vi "LinearSystemLoop_DiffDrv_Pack_Ctrl.vi"(4 "Max Control Effort":dbl=12.0, 6 "Right Vel Ctrl Tol m/s":dbl=0.04, 7 "Left Vel Model Std Dev m/s":dbl=0.1, 8 "Left Vel Ctrl Tol m/s":dbl=0.04, 9 "Right Vel Meas Std Dev m/s":dbl=0.03, 10 "Left Vel Meas Std Dev m/s":dbl=0.03, 11 "Right Vel Model Std Dev m/s":dbl=0.1) -> (3 "LinearSystemLoop_DiffDrv_Ctrl_Params":T1={"Left Vel Model Std Dev m/s"=0.0, "Left Vel Meas Std Dev m/s"=0.0, "Left Vel Ctrl Tol m/s"=0.0, "Max Control Effort"=0.0, "Right Vel Ctrl Tol m/s"=0.8, "Right Vel Meas Std Dev m/s"=0.02, "Right Vel Model Std Dev m/s"=0.0})   [LabVIEW 2019, in "Trajectory_Library.lvlib"]
uses:
  Trajectory_Library.lvlib
  TypeDef/LINEAR_SYSTEM_LOOP_DIFF_DRV_CTRL_PARAMS.CTL
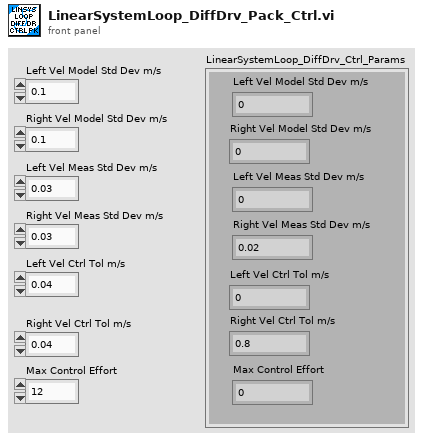
[diagram p1: front panel]
types:
  T1 = typedef "Trajectory_Library.lvlib/LINEAR_SYSTEM_LOOP_DIFF_DRV_CTRL_PARAMS.CTL" = cluster{"Left Vel Model Std Dev m/s":dbl, "Left Vel Meas Std Dev m/s":dbl, "Left Vel Ctrl Tol m/s":dbl, "Max Control Effort":dbl, "Right Vel Ctrl Tol m/s":dbl, "Right Vel Meas Std Dev m/s":dbl, "Right Vel Model Std Dev m/s":dbl}
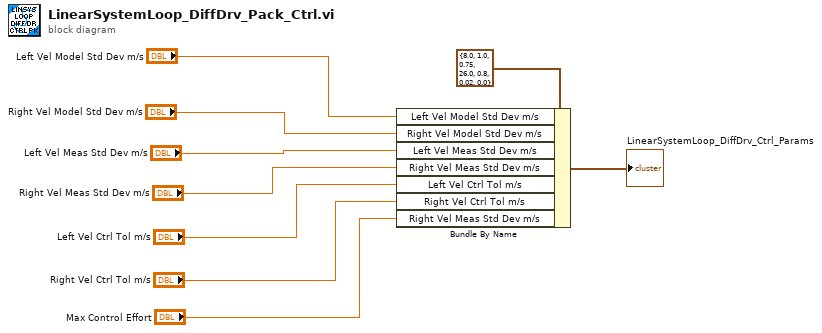
[diagram p0: block diagram]
diagram:
  n1 = Bundle By Name(cluster=T1 {"Left Vel Model Std Dev m/s"=8.0, "Left Vel Meas Std Dev m/s"=1.0, "Left Vel Ctrl Tol m/s"=0.75, "Max Control Effort"=26.0, "Right Vel Ctrl Tol m/s"=0.8, "Right Vel Meas Std Dev m/s"=0.02, "Right Vel Model Std Dev m/s"=0.0} ("DCMotorSim_Model _Params"), "Left Vel Model Std Dev m/s"="Left Vel Model Std Dev m/s", "Right Vel Model Std Dev m/s"="Right Vel Model Std Dev m/s", "Left Vel Meas Std Dev m/s"="Left Vel Meas Std Dev m/s", "Right Vel Meas Std Dev m/s"="Right Vel Meas Std Dev m/s", "Left Vel Ctrl Tol m/s"="Left Vel Ctrl Tol m/s", "Right Vel Ctrl Tol m/s"="Right Vel Ctrl Tol m/s", "Right Vel Meas Std Dev m/s"="Max Control Effort") -> (→"LinearSystemLoop_DiffDrv_Ctrl_Params":T1)
